vi "main.vi"() -> ()   [LabVIEW 2014]
uses:
  select.ctl
  Data.ctl
  <vilib>/Utility/miscctls.llb/LVBoundsTypeDef.ctl
panel:
  out "9":picture
  out "8":picture
  out "7":picture
  out "6":picture
  out "5":picture
  out "4":picture
  out "3":picture
  out "2":picture
  out "1":picture
  out "zero":picture
  out "ResultsAcumulado":string[][][](array[string])
  out "Listbox":i32(listbox)
  in  "Choose":string(combo)="luck"
  in  "Name":string
  in  "Exit":bool
  in  "Go":bool
  in  "ErrorIn":errorcluster
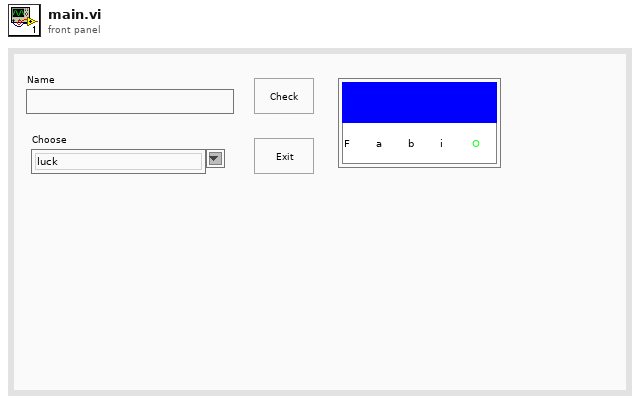
[diagram p1: front panel]
types:
  T1 = typedef "Data.ctl" = cluster{"Name":string, "Singles&Doubles":string[], "Results":string[][], "SinglesInOrder":string[], "DoublesInOrder":string[], "Option":string, "AllLetters":string[], "ByLuck":string, "SIndex":string[], "DIndex":string[], "ListOfNames":string[], "Cycles":cluster{"Laps":i32, "Counter":i32}, "Array":cluster{"AllLetters":string[], "ByLuck":string, "Option":string}[], "all":string[][], "all 2":string[][][], "WhichAndWhere":i32[], "Array 2":cluster{"AllLetters":string[], "ByLuck":string}[], "Chosen":string, "OptionForLuck":string, "ResultsAcumulado":string[][][]}
  T2 = typedef "select.ctl" = enum16{"init", "idle", "Segregate", "Select", "Singles&Doubles", "SearchForElements", "Display", "PutInOrder", "OptionToSelect", "Selected", "ChooseByLuck", "PrepareToShowByLuck", "PrepareToShowSelected", "Show", "ShowOnce"}
  T3 = cluster{"AllLetters":string[], "ByLuck":string}[]
  T4 = cluster{"AllLetters":string[], "ByLuck":string, "Option":string}[]
  T5 = typedef "LVBoundsTypeDef.ctl" = cluster{"Width":u32, "Height":u32}
  T6 = typedef "imagedata.ctl" = cluster{"image type":i32, "image depth":i32, "image":u8[], "mask":u8[], "colors":u32[], "Rectangle":cluster{"left":i16, "top":i16, "right":i16, "bottom":i16}}
  T7 = cluster{"AllLetters":string[], "ByLuck":string, "OptionForLuck":string}
  T8 = cluster{"AllLetters":string[], "ByLuck":string, "OptionForLuck":string}[]
  T9 = cluster{"AllLetters":string[], "Chosen":string}[]
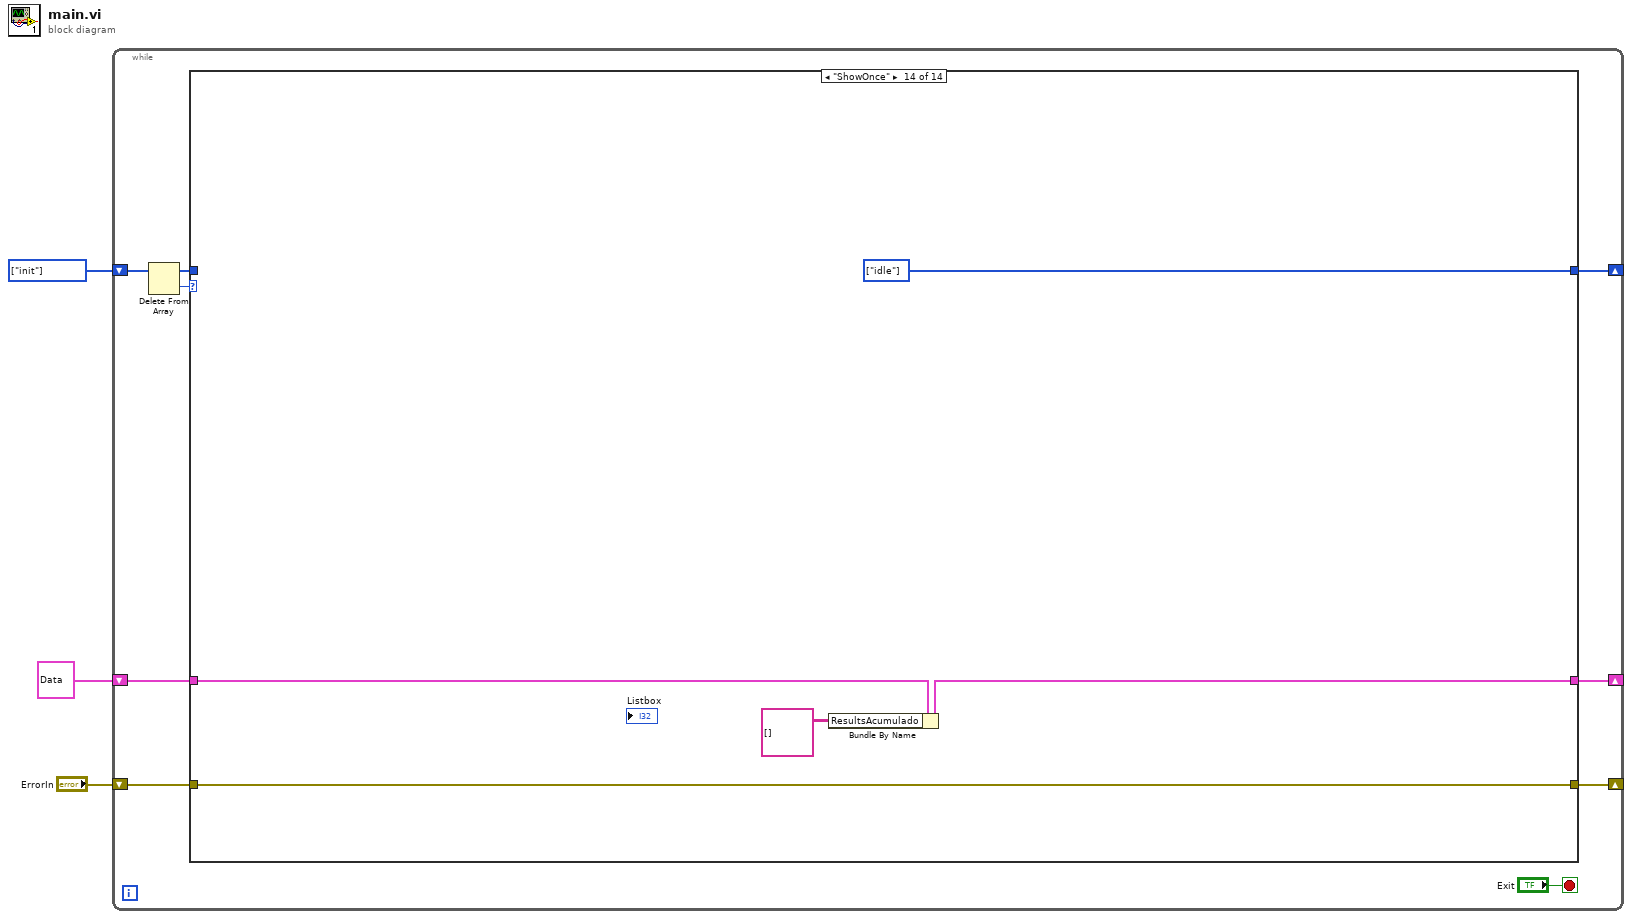
[diagram p0: block diagram]
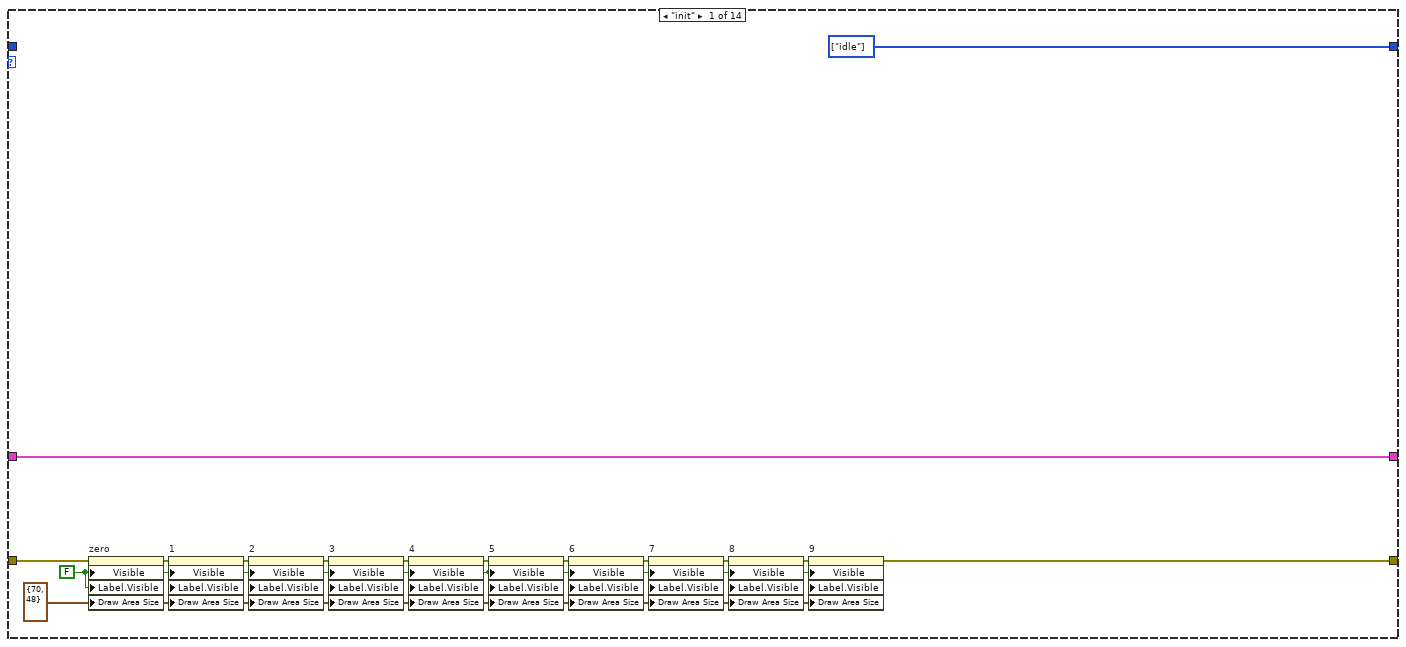
[diagram p2: hidden frame]
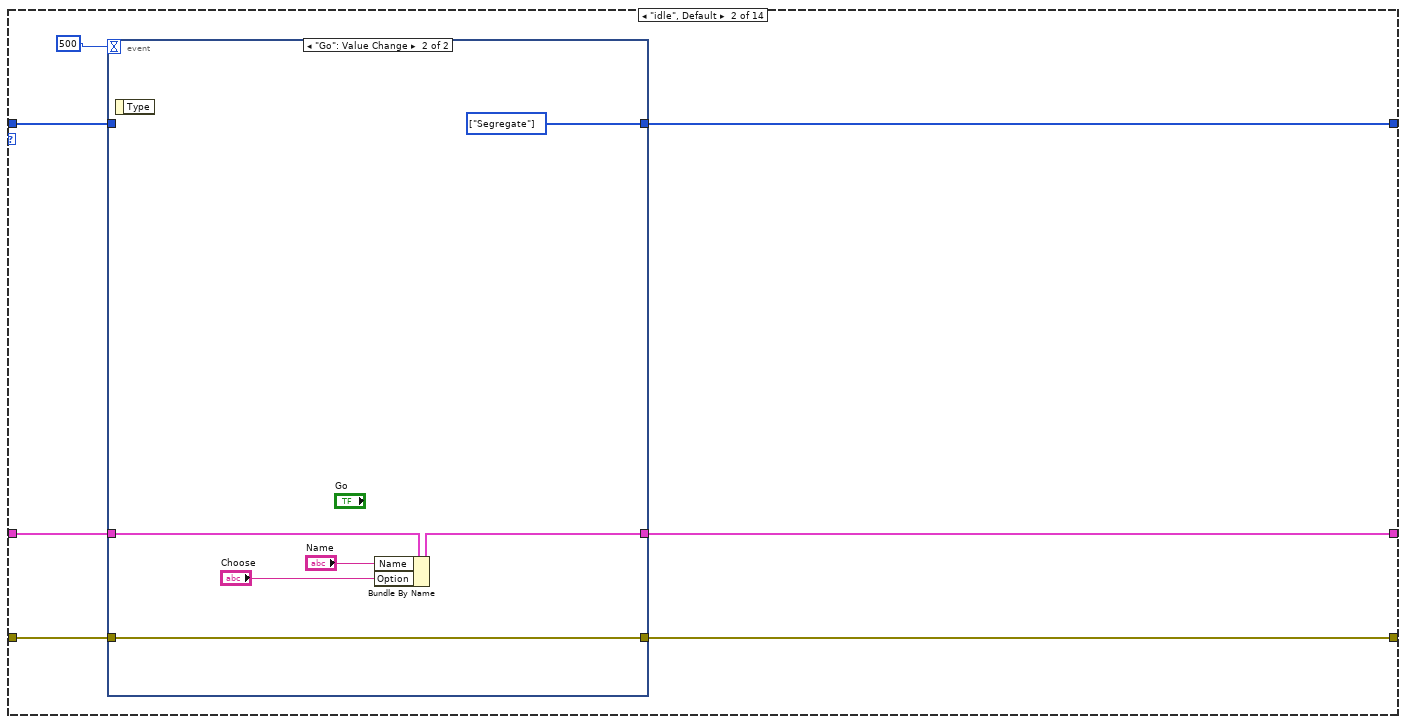
[diagram p3: hidden frame]
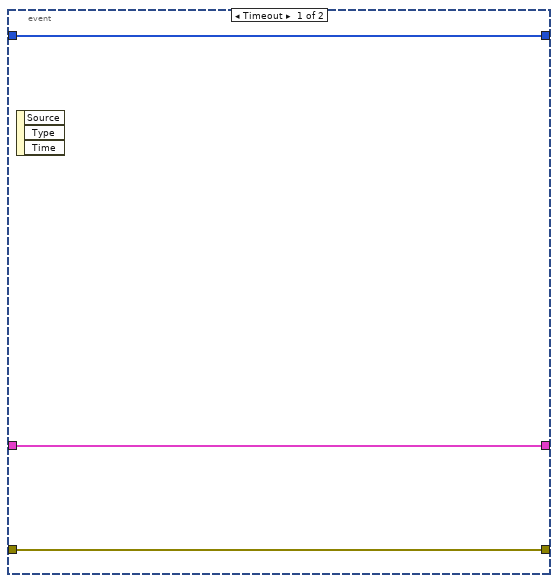
[diagram p4: hidden frame]
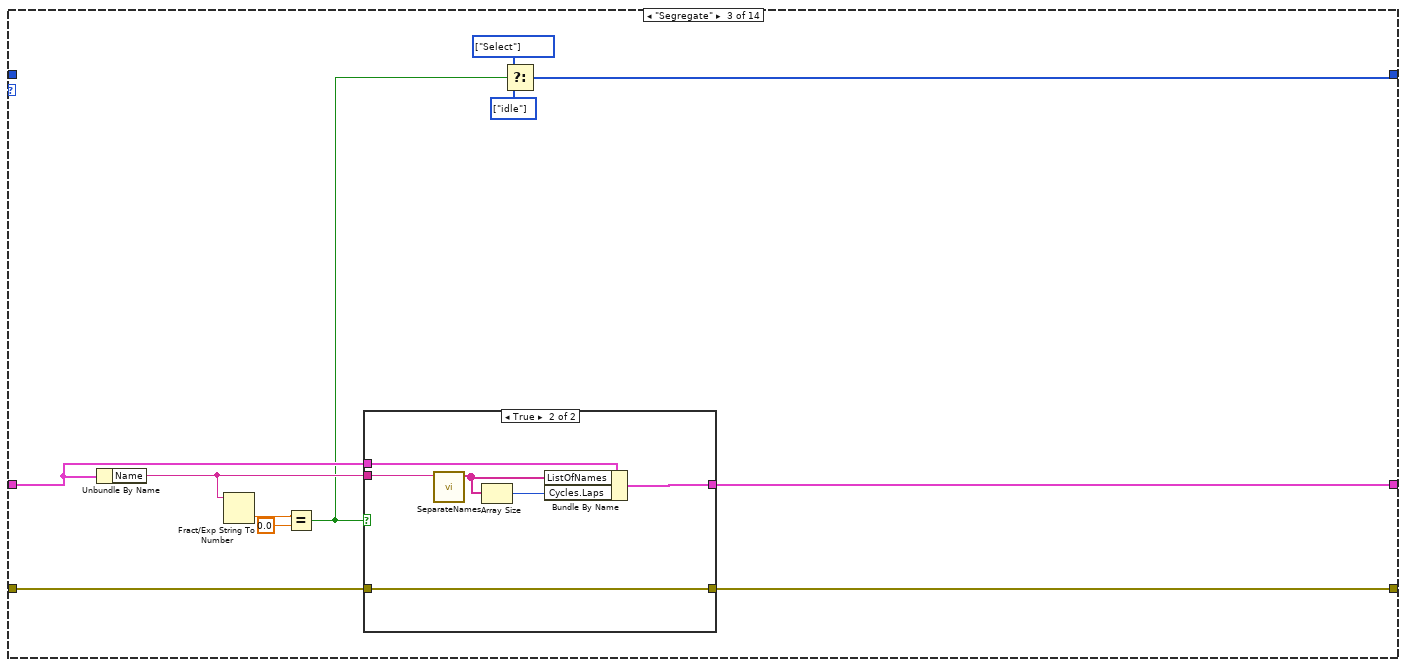
[diagram p5: hidden frame]
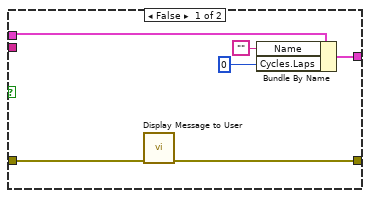
[diagram p6: hidden frame]
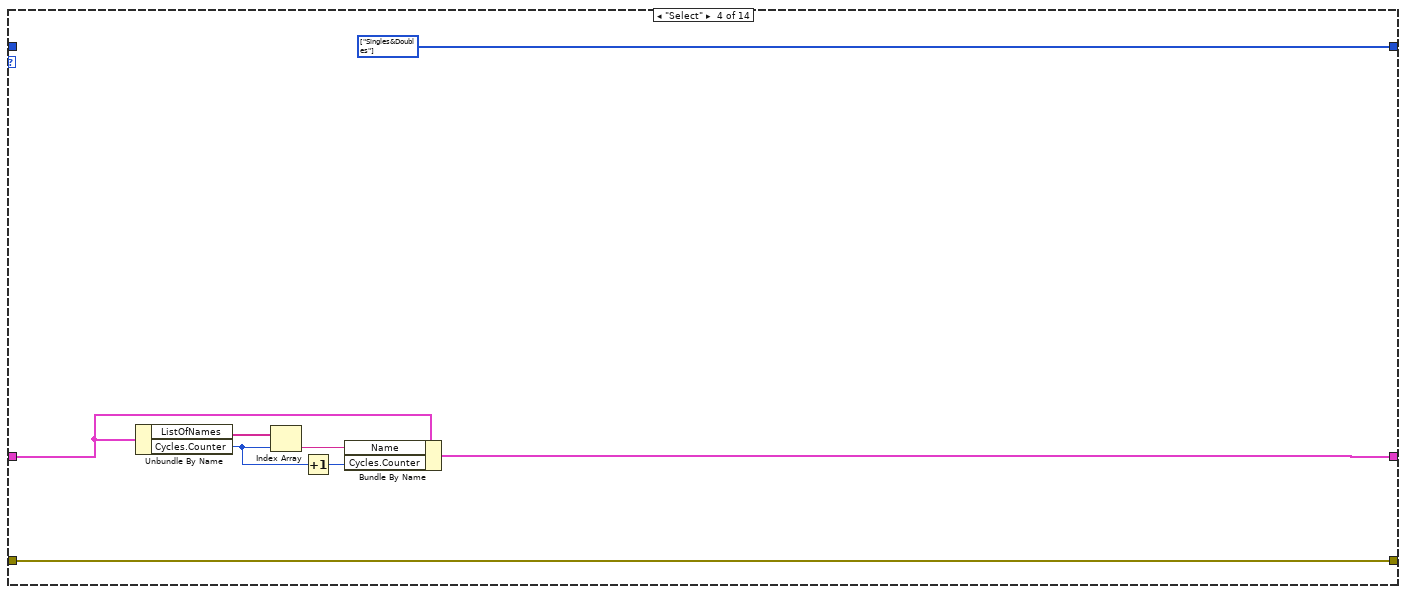
[diagram p7: hidden frame]
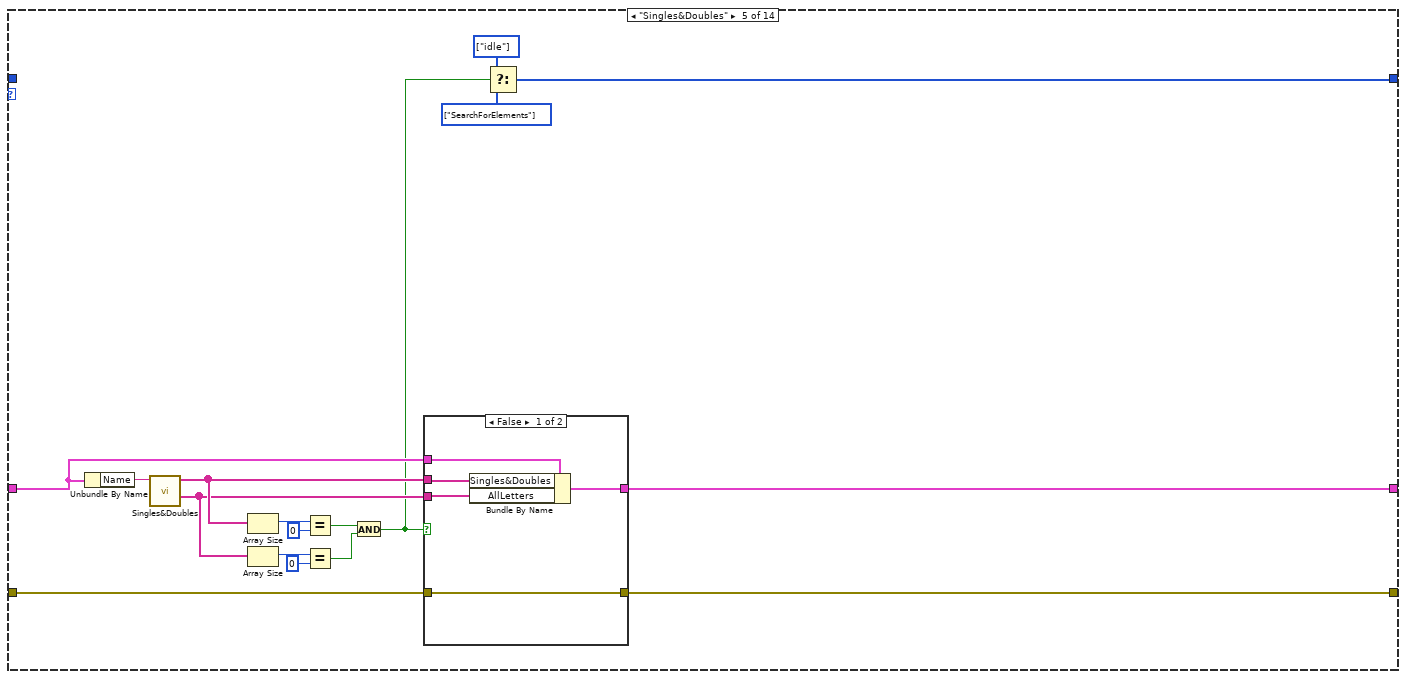
[diagram p8: hidden frame]
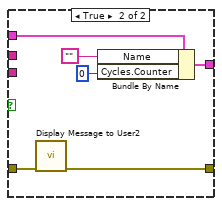
[diagram p9: hidden frame]
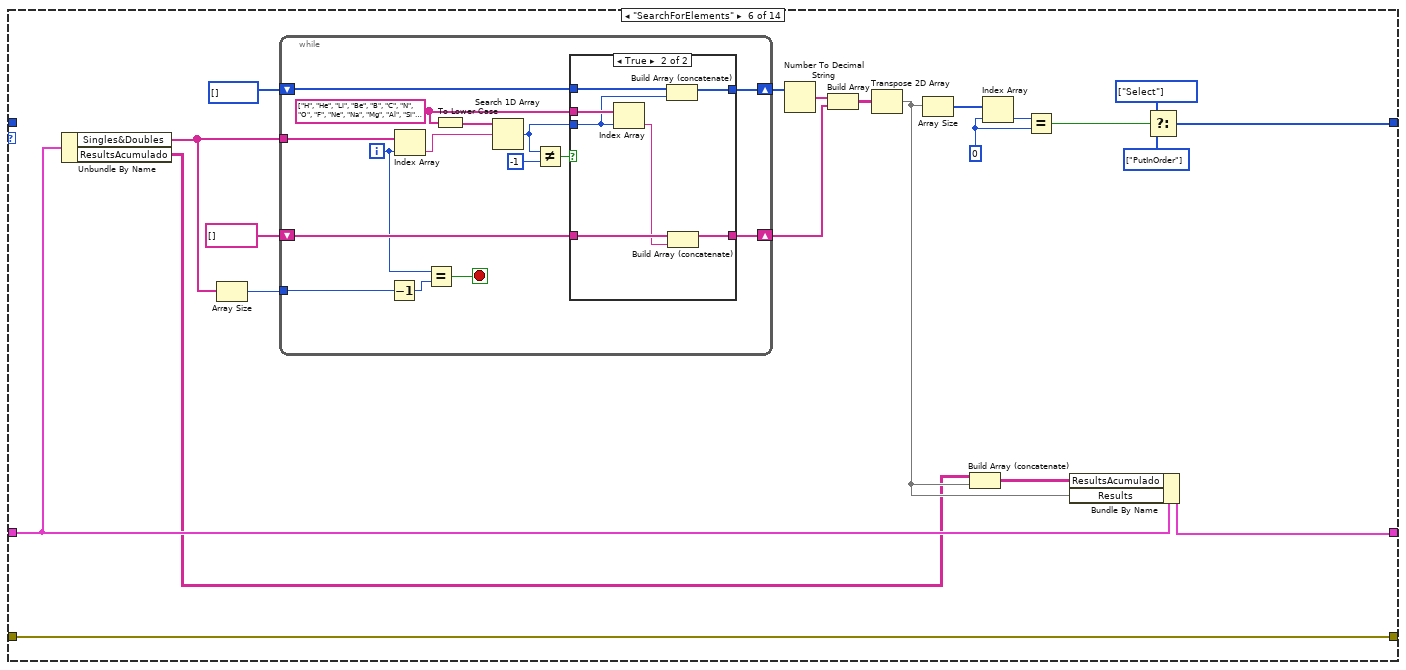
[diagram p10: hidden frame]
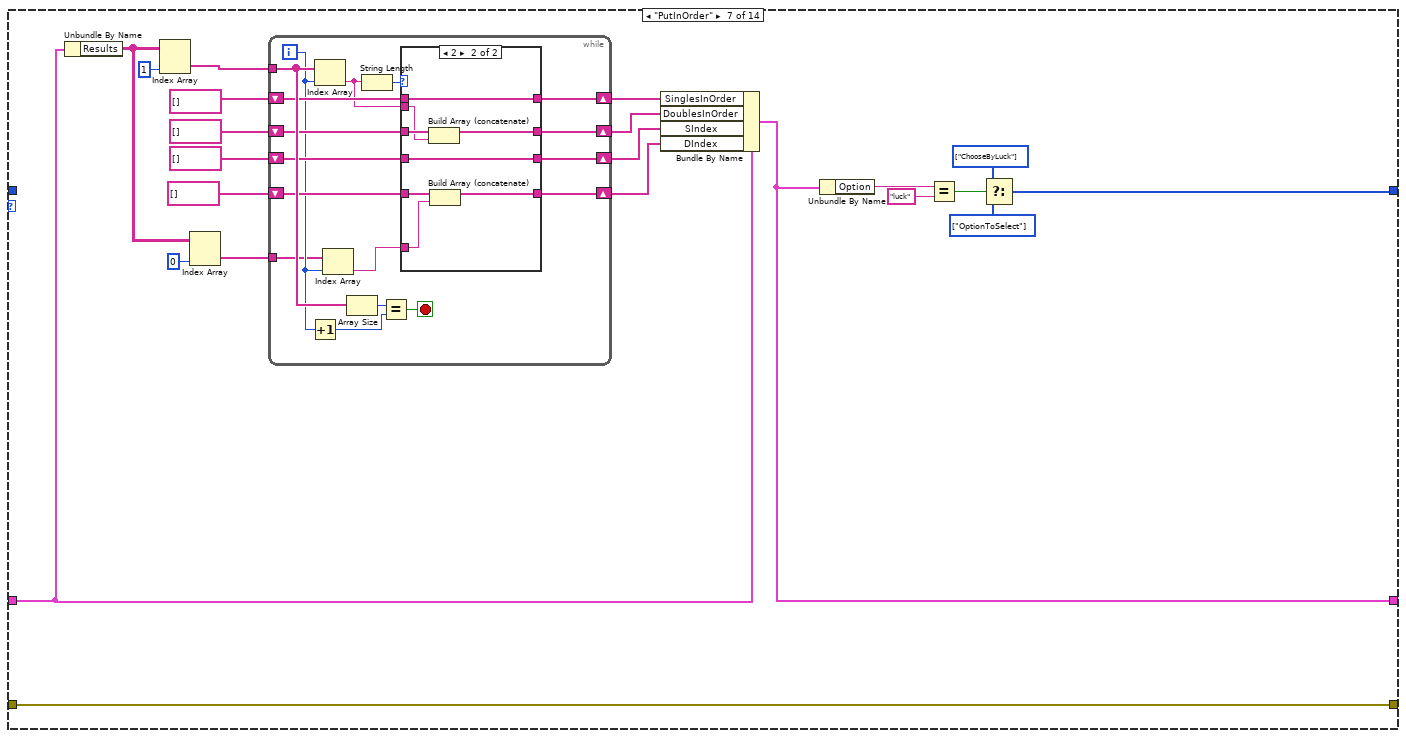
[diagram p12: hidden frame]
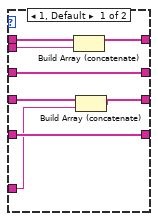
[diagram p13: hidden frame]
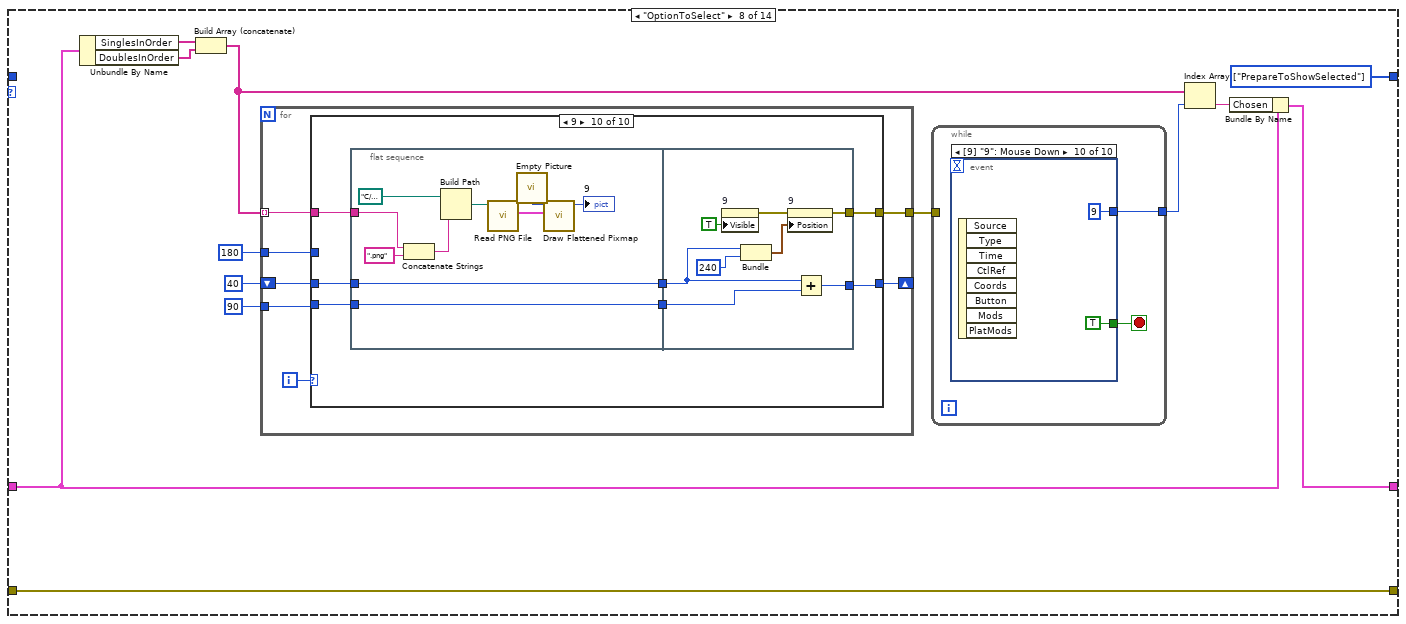
[diagram p14: hidden frame]
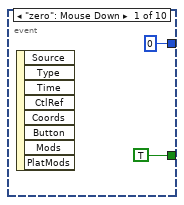
[diagram p15: hidden frame]
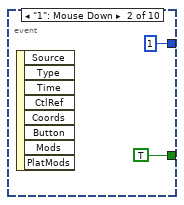
[diagram p16: hidden frame]
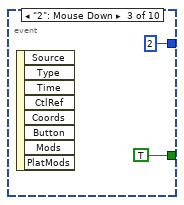
[diagram p17: hidden frame]
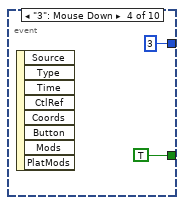
[diagram p18: hidden frame]
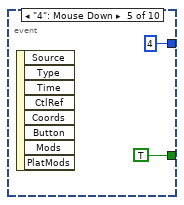
[diagram p19: hidden frame]
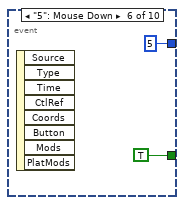
[diagram p20: hidden frame]
diagram:
  w3 = T2[] [enum."init"] items=["init", "idle", "Segregate", "Select", "Singles&Doubles", "SearchForElements", "Display", "PutInOrder", "OptionToSelect", "Selected", "ChooseByLuck", "PrepareToShowByLuck", "PrepareToShowSelected", "Show", "ShowOnce"]
  n1 = while {
    shift-right: [w9] -> _
    shift-left: w3 -> [w12]
    shift-right: [w7] -> _
    shift-left: T1 {"Name"="", "Singles&Doubles"=[], "Results"=[], "SinglesInOrder"=[], "DoublesInOrder"=[], "Option"="", "AllLetters"=[], "ByLuck"="", "SIndex"=[], "DIndex"=[], "ListOfNames"=[], "Cycles"={"Laps"=0, "Counter"=0}, "Array"=[], "all"=[], "all 2"=[], "WhichAndWhere"=[], "Array 2"=[], "Chosen"="", "OptionForLuck"="", "ResultsAcumulado"=[]} -> [w8]
    shift-right: [w6] -> _
    shift-left: "ErrorIn" -> [w5]
    stop <- "Exit" stop-if-true
    n2 = Delete From Array(array=w12) -> (deleted portion=w11:T2, array with subset deleted=w10:T2[])  [unwired: 2 in]
    n3 = case shown="\"ShowOnce\"" w11 {
      tunnel: w10 -> [_ w30 _ _ _ _ _ _ _ _ _ _ _ _]
      tunnel: [w14 w34 w48 w68 w75 w107 w154 w214 w505 w537 w553 w592 w626 w647] -> w9
      tunnel: w8 -> [w15 w33 w54 w73 w91 w120 w168 w211 w508 w536 w555 w588 w622 w646]
      tunnel: [w15 w32 w53 w69 w90 w119 w153 w210 w507 w535 w552 w584 w621 w645] -> w7
      tunnel: [w17 w28 w46 w67 w79 w123 w169 w215 w506 w540 w554 w601 w602 w643] -> w6
      tunnel: w5 -> [w16 w31 w47 w67 w80 w123 w169 w215 w506 w540 w554 w601 w612 w643]
      frame "init" {
        w13 = T5 {"Width"=70, "Height"=48} ("Bounds")
        w14 = T2[] [enum."idle"] items=["init", "idle", "Segregate", "Select", "Singles&Doubles", "SearchForElements", "Display", "PutInOrder", "OptionToSelect", "Selected", "ChooseByLuck", "PrepareToShowByLuck", "PrepareToShowSelected", "Show", "ShowOnce"] ("f")
        w18 = FALSE
        n4 = property on="zero" class="Pict"(error in=w16, "Visible"=w18, "Label.Visible"=w18, "Draw Area Size"=w13) -> (error out=w19:errorcluster)  [unwired: 1 in, 1 out]
        n5 = property on="1" class="Pict"(error in=w19, "Visible"=w18, "Label.Visible"=w18, "Draw Area Size"=w13) -> (error out=w20:errorcluster)  [unwired: 1 in, 1 out]
        n6 = property on="2" class="Pict"(error in=w20, "Visible"=w18, "Label.Visible"=w18, "Draw Area Size"=w13) -> (error out=w21:errorcluster)  [unwired: 1 in, 1 out]
        n7 = property on="3" class="Pict"(error in=w21, "Visible"=w18, "Label.Visible"=w18, "Draw Area Size"=w13) -> (error out=w22:errorcluster)  [unwired: 1 in, 1 out]
        n8 = property on="4" class="Pict"(error in=w22, "Visible"=w18, "Label.Visible"=w18, "Draw Area Size"=w13) -> (error out=w23:errorcluster)  [unwired: 1 in, 1 out]
        n9 = property on="5" class="Pict"(error in=w23, "Visible"=w18, "Label.Visible"=w18, "Draw Area Size"=w13) -> (error out=w24:errorcluster)  [unwired: 1 in, 1 out]
        n10 = property on="6" class="Pict"(error in=w24, "Visible"=w18, "Label.Visible"=w18, "Draw Area Size"=w13) -> (error out=w25:errorcluster)  [unwired: 1 in, 1 out]
        n11 = property on="7" class="Pict"(error in=w25, "Visible"=w18, "Label.Visible"=w18, "Draw Area Size"=w13) -> (error out=w26:errorcluster)  [unwired: 1 in, 1 out]
        n12 = property on="8" class="Pict"(error in=w26, "Visible"=w18, "Label.Visible"=w18, "Draw Area Size"=w13) -> (error out=w27:errorcluster)  [unwired: 1 in, 1 out]
        n13 = property on="9" class="Pict"(error in=w27, "Visible"=w18, "Label.Visible"=w18, "Draw Area Size"=w13) -> (error out=w17:errorcluster)  [unwired: 1 in, 1 out]
      }
      frame "idle", Default {
        n14 = event shown="[1] \"Go\": Value Change" {
          selector: _ -> [_ _]
          dyn-events: _ -> [_ _]
          timeout: 500 -> [_ _]
          tunnel: w30 -> [w37 _]
          tunnel: [w37 w42] -> w34
          tunnel: [w36 w40] -> w32
          tunnel: w33 -> [w36 w41]
          tunnel: [w35 w43] -> w28
          tunnel: w31 -> [w35 w43]
          event Timeout {
            n15 = event-data() -> ()  [unwired: 1 in, 3 out]
          }
          event "Go": Value Change {
            w42 = T2[] [enum."Segregate"] items=["init", "idle", "Segregate", "Select", "Singles&Doubles", "SearchForElements", "Display", "PutInOrder", "OptionToSelect", "Selected", "ChooseByLuck", "PrepareToShowByLuck", "PrepareToShowSelected", "Show", "ShowOnce"]
            n16 = event-data() -> ()  [unwired: 1 in, 1 out]
            n17 = Bundle By Name(cluster=w41, "Name"="Name", "Option"="Choose") -> (w40:T1)
          }
        }
      }
      frame "Segregate" {
        w45 = T2[] [enum."idle"] items=["init", "idle", "Segregate", "Select", "Singles&Doubles", "SearchForElements", "Display", "PutInOrder", "OptionToSelect", "Selected", "ChooseByLuck", "PrepareToShowByLuck", "PrepareToShowSelected", "Show", "ShowOnce"]
        w44 = T2[] [enum."Select"] items=["init", "idle", "Segregate", "Select", "Singles&Doubles", "SearchForElements", "Display", "PutInOrder", "OptionToSelect", "Selected", "ChooseByLuck", "PrepareToShowByLuck", "PrepareToShowSelected", "Show", "ShowOnce"]
        n18 = Unbundle By Name(w54) -> ("Name"=w52:string)
        n19 = Fract/Exp String To Number(string=w52) -> (number=w51:dbl)  [unwired: 3 in, 1 out]
        n20 = Equal?(x=w51, y=0.0) -> (x = y?=w49:bool)
        n21 = case shown="True" w49 {
          tunnel: w52 -> [_ w66]
          tunnel: w54 -> [w58 w65]
          tunnel: [w57 w62] -> w53
          tunnel: w47 -> [w60 w61]
          tunnel: [w59 w61] -> w46
          frame False {
            n22 = call "Display Message to User"("error in (no error)"=w60) -> ("error out"=w59:errorcluster)  [unwired: 9 in, 1 out]
            n23 = Bundle By Name(cluster=w58, "Name"="", "Cycles.Laps"=0) -> (w57:T1)
          }
          frame True {
            n24 = call "SeparateNames.vi"("CompleteName"=w66) -> ("SeparateWords"=w63:string[])  [unwired: 10 in]
            n25 = Array Size(array=w63) -> (size(s)=w64:i32)
            n26 = Bundle By Name(cluster=w65, "ListOfNames"=w63, "Cycles.Laps"=w64) -> (w62:T1)
          }
        }
        n27 = Select(t=w44, s=w49, f=w45) -> (s? t:f=w48:T2[])
      }
      frame "Select" {
        w68 = T2[] [enum."Singles&Doubles"] items=["init", "idle", "Segregate", "Select", "Singles&Doubles", "SearchForElements", "Display", "PutInOrder", "OptionToSelect", "Selected", "ChooseByLuck", "PrepareToShowByLuck", "PrepareToShowSelected", "Show", "ShowOnce"]
        n28 = Unbundle By Name(w73) -> ("ListOfNames"=w74:string[], "Cycles.Counter"=w71:i32)
        n29 = Index Array(array=w74, index=w71) -> (element=w70:string)
        n30 = Increment(x=w71) -> (x+1=w72:i32)
        n31 = Bundle By Name(cluster=w73, "Name"=w70, "Cycles.Counter"=w72) -> (w69:T1)
      }
      frame "Singles&Doubles" {
        w76 = T2[] [enum."idle"] items=["init", "idle", "Segregate", "Select", "Singles&Doubles", "SearchForElements", "Display", "PutInOrder", "OptionToSelect", "Selected", "ChooseByLuck", "PrepareToShowByLuck", "PrepareToShowSelected", "Show", "ShowOnce"]
        w77 = T2[] [enum."SearchForElements"] items=["init", "idle", "Segregate", "Select", "Singles&Doubles", "SearchForElements", "Display", "PutInOrder", "OptionToSelect", "Selected", "ChooseByLuck", "PrepareToShowByLuck", "PrepareToShowSelected", "Show", "ShowOnce"]
        n32 = Unbundle By Name(w91) -> ("Name"=w89:string)
        n33 = call "Singles&Doubles.vi"("Name"=w89) -> ("AllLetters"=w87:string[], "Singles&Doubles"=w88:string[])  [unwired: 9 in]
        n34 = Array Size(array=w88) -> (size(s)=w86:i32)
        n35 = Array Size(array=w87) -> (size(s)=w85:i32)
        n36 = Equal?(x=w86, y=0) -> (x = y?=w82:bool)
        n37 = Equal?(x=w85, y=0) -> (x = y?=w81:bool)
        n38 = And(x=w82, y=w81) -> (x .and. y?=w78:bool)
        n39 = case shown="False" w78 {
          tunnel: w91 -> [w96 w100]
          tunnel: [w95 w99] -> w90
          tunnel: w88 -> [w94 _]
          tunnel: w87 -> [w93 _]
          tunnel: w80 -> [w92 w102]
          tunnel: [w92 w101] -> w79
          frame False {
            n40 = Bundle By Name(cluster=w96, "Singles&Doubles"=w94, "AllLetters"=w93) -> (w95:T1)
          }
          frame True {
            n41 = call "Display Message to User2"("error in (no error)"=w102) -> ("error out"=w101:errorcluster)  [unwired: 9 in, 1 out]
            n42 = Bundle By Name(cluster=w100, "Name"="", "Cycles.Counter"=0) -> (w99:T1)
          }
        }
        n43 = Select(t=w76, s=w78, f=w77) -> (s? t:f=w75:T2[])
      }
      frame "SearchForElements" {
        w106 = T2[] [enum."Select"] items=["init", "idle", "Segregate", "Select", "Singles&Doubles", "SearchForElements", "Display", "PutInOrder", "OptionToSelect", "Selected", "ChooseByLuck", "PrepareToShowByLuck", "PrepareToShowSelected", "Show", "ShowOnce"] ("t")
        w110 = 0
        w108 = T2[] [enum."PutInOrder"] items=["init", "idle", "Segregate", "Select", "Singles&Doubles", "SearchForElements", "Display", "PutInOrder", "OptionToSelect", "Selected", "ChooseByLuck", "PrepareToShowByLuck", "PrepareToShowSelected", "Show", "ShowOnce"]
        n44 = Unbundle By Name(w120) -> ("Singles&Doubles"=w118:string[], "ResultsAcumulado"=w103:string[][][])
        n45 = Array Size(array=w118) -> (size(s)=w121:i32)
        n46 = while {
          tunnel: w118 -> [w133]
          shift-right: [w135] -> w114
          shift-left: string[] [] -> [w134]
          tunnel: w121 -> [w127]
          shift-right: [w125] -> w113
          shift-left: i32[] [] -> [w124]
          i -> [w131]
          stop <- w130 stop-if-true
          w126 = string[] ["H", "He", "Li", "Be", "B", "C", "N", "O", "F", "Ne", "Na", "Mg", "Al", "Si", "P", "S", "Cl", "Ar", "K", "Ca", "Sc", "Ti", "V", "Cr", "Mn", "Fe", "Co", "Ni", "Cu", "Zn", "Ga", "Ge", "As", "Se", "Br", "Kr", "Rb", "Sr", "Y", "Zr", "Nb", "Mo", "Tc", "Ru", "Rh", "Pd", "Ag", "Cd", "In", "Sn", "Sb", "Te", "I", "Xe", "Cs", "Ba", "La", "Ce", "Pr", "Nd", "Pm", "Sm", "Eu", "Gd", "Tb", "Dy", "Ho", "Er", "Tm", "Yb", "Lu", "Hf", "Ta", "W", "Re", "Os", "Ir", "Pt", "Au", "Hg", "Tl", "Pb", "Bi", "Po", "At", "Rn", "Fr", "Ra", "Ac", "Th", "Pa", "U", "Np", "Pu", "Am", "Cm", "Bk", "Cf", "Es", "Fm", "Md", "No", "Lr", "Rf", "Db", "Sg", "Bh", "Hs", "Mt"]
          n47 = Decrement(x=w127) -> (x-1=w128:i32)
          n48 = Index Array(array=w133, index=w131) -> (element=w138:string)
          n49 = Equal?(x=w131, y=w128) -> (x = y?=w130:bool)
          n50 = To Lower Case(string=w126) -> (all lower case string=w129:string[])
          n51 = Search 1D Array(1D array=w129, element=w138) -> (index of element=w132:i32)  [unwired: 1 in]
          n52 = Not Equal?(x=w132, y=-1) -> (x != y?=w136:bool)
          n53 = case shown="True" w136 {
            tunnel: [w140 w144] -> w135
            tunnel: w134 -> [w140 w147]
            tunnel: w126 -> [_ w146]
            tunnel: w132 -> [_ w141]
            tunnel: [w139 w143] -> w125
            tunnel: w124 -> [w139 w142]
            frame False {
            }
            frame True {
              n54 = Index Array(array=w146, index=w141) -> (element=w145:string)
              n55 = Build Array (concatenate)(w142, w141) -> (w143:i32[])
              n56 = Build Array (concatenate)(w147, w145) -> (w144:string[])
            }
          }
        }
        n57 = Number To Decimal String(number=w113) -> (decimal integer string=w116:string[])  [unwired: 1 in]
        n58 = Build Array(w116, w114) -> (w115:string[][])
        n59 = Transpose 2D Array(2D array=w115) -> (transposed array=w104:string[][])
        n60 = Array Size(array=w104) -> (size(s)=w112:i32[])
        n61 = Build Array (concatenate)(w103, w104) -> (w105:string[][][])
        n62 = Index Array(array=w112, index=w110) -> (element=w111:i32)
        n63 = Equal?(x=w111, y=w110) -> (x = y?=w109:bool)
        n64 = Bundle By Name(cluster=w120, "ResultsAcumulado"=w105, "Results"=w104) -> (w119:T1)
        n65 = Select(t=w106, s=w109, f=w108) -> (s? t:f=w107:T2[])
      }
      frame "PutInOrder" {
        w149 = T2[] [enum."OptionToSelect"] items=["init", "idle", "Segregate", "Select", "Singles&Doubles", "SearchForElements", "Display", "PutInOrder", "OptionToSelect", "Selected", "ChooseByLuck", "PrepareToShowByLuck", "PrepareToShowSelected", "Show", "ShowOnce"]
        w150 = T2[] [enum."ChooseByLuck"] items=["init", "idle", "Segregate", "Select", "Singles&Doubles", "SearchForElements", "Display", "PutInOrder", "OptionToSelect", "Selected", "ChooseByLuck", "PrepareToShowByLuck", "PrepareToShowSelected", "Show", "ShowOnce"]
        n66 = Unbundle By Name(w168) -> ("Results"=w156:string[][])
        n67 = Index Array(array=w156, index (col)=1 ("disabled index (col)")) -> (element=w158:string[])  [unwired: 1 in]
        n68 = Index Array(array=w156, index (col)=0 ("disabled index (col)")) -> (element=w155:string[])  [unwired: 1 in]
        n69 = while {
          tunnel: w158 -> [w186]
          shift-right: [w183] -> w165
          shift-left: string[] [] -> [w182]
          shift-right: [w180] -> w164
          shift-left: string[] [] -> [w181]
          shift-right: [w178] -> w161
          shift-left: string[] [] -> [w179]
          shift-right: [w176] -> w160
          shift-left: string[] [] -> [w177]
          tunnel: w155 -> [w173]
          i -> [w174]
          stop <- w171 stop-if-true
          n70 = Increment(x=w174) -> (x+1=w184:i32)
          n71 = Index Array(array=w186, index=w174) -> (element=w175:string)
          n72 = Index Array(array=w173, index=w174) -> (element=w172:string)
          n73 = Array Size(array=w186) -> (size(s)=w185:i32)
          n74 = String Length(string=w175) -> (length=w170:i32)
          n75 = Equal?(x=w185, y=w184) -> (x = y?=w171:bool)
          n76 = case shown="2" w170 {
            tunnel: [w192 w202] -> w183
            tunnel: w182 -> [w194 w202]
            tunnel: w181 -> [w193 w200]
            tunnel: [w193 w201] -> w180
            tunnel: w179 -> [w191 w197]
            tunnel: [w190 w197] -> w178
            tunnel: w177 -> [w189 w198]
            tunnel: [w189 w199] -> w176
            tunnel: w175 -> [w188 w196]
            tunnel: w172 -> [w187 w195]
            frame 1, Default {
              n77 = Build Array (concatenate)(w194, w188) -> (w192:string[])
              n78 = Build Array (concatenate)(w191, w187) -> (w190:string[])
            }
            frame 2 {
              n79 = Build Array (concatenate)(w200, w196) -> (w201:string[])
              n80 = Build Array (concatenate)(w198, w195) -> (w199:string[])
            }
          }
        }
        n81 = Bundle By Name(cluster=w168, "SinglesInOrder"=w165, "DoublesInOrder"=w164, "SIndex"=w161, "DIndex"=w160) -> (w153:T1)
        n82 = Unbundle By Name(w153) -> ("Option"=w152:string)
        n83 = Equal?(x=w152, y="luck") -> (x = y?=w148:bool)
        n84 = Select(t=w150, s=w148, f=w149) -> (s? t:f=w154:T2[])
      }
      frame "OptionToSelect" {
        w214 = T2[] [enum."PrepareToShowSelected"] items=["init", "idle", "Segregate", "Select", "Singles&Doubles", "SearchForElements", "Display", "PutInOrder", "OptionToSelect", "Selected", "ChooseByLuck", "PrepareToShowByLuck", "PrepareToShowSelected", "Show", "ShowOnce"] ("f")
        n85 = Unbundle By Name(w211) -> ("SinglesInOrder"=w213:string[], "DoublesInOrder"=w212:string[])
        n86 = Build Array (concatenate)(w213, w212) -> (w204:string[])
        n87 = for {
          tunnel: w204 -> [w239] mode=indexing
          shift-right: [w243] -> _
          shift-left: 40 -> [w244]
          tunnel: 90 ("y") -> [w241]
          tunnel: [w240] -> w206
          tunnel: 180 -> [w238]
          i -> [w242]
          n88 = case shown="9" w242 {
            tunnel: w239 -> [w252 w280 w308 w336 w364 w389 w411 w434 w459 w485]
            tunnel: w244 -> [w251 w279 w307 w335 w363 _ _ w433 w458 w484]
            tunnel: [w250 w278 w306 w334 w362 w388 w410 w432 w457 w483] -> w243
            tunnel: w241 -> [w248 w276 w305 w333 w361 w387 w409 w431 w456 w482]
            tunnel: [w247 w275 w303 w331 w359 w385 w407 w429 w454 w480] -> w240
            tunnel: w238 -> [w245 w273 w302 w330 w358 _ _ _ _ _]
            frame 0, Default {
              n89 = flat-sequence {
                tunnel: w252 -> [w257]
                tunnel: [w259] -> w253
                tunnel: w251 -> [w259]
                tunnel: [w255] -> w249
                tunnel: w248 -> [w255]
                tunnel: [w254] -> w246
                tunnel: w245 -> [w254]
                tunnel: w253 -> [w266]
                tunnel: [w271] -> w250
                tunnel: w249 -> [w270]
                tunnel: [w269] -> w247
                tunnel: w246 -> [w265]
                frame #0 {
                  n90 = Concatenate Strings(w257, ".png" ("string")) -> (w258:string)
                  n91 = Build Path(base path=path "C:/Users/beck.to.beck/Documents/LabVIEW Data/BrBa/elements", name or relative path=w258) -> (appended path=w262:path)
                  n92 = call <vilib>:"Read PNG File.vi"("path to PNG file"=w262) -> ("image data"=w261:T6)  [unwired: 8 in, 2 out]
                  n93 = call "Empty Picture"() -> ("empty picture"=w263:picture)
                  n94 = call <vilib>:"Draw Flattened Pixmap.vi"("image data"=w261, "picture"=w263) -> ("new picture"=→"zero":picture)  [unwired: 7 in]
                }
                frame #1 {
                  n95 = property on="zero" class="Pict"("Visible"=TRUE) -> (error out=w267:errorcluster)  [unwired: 2 in, 1 out]
                  n96 = Bundle(w266, w265) -> (w272:cluster{i32, i32})  [unwired: 1 in]
                  n97 = property on="zero" class="Pict"(error in=w267, "Position"=w272) -> (error out=w269:errorcluster)  [unwired: 1 in, 1 out]
                  n98 = Add(x=w266, y=w270) -> (x+y=w271:i32)
                }
              }
            }
            frame 1 {
              n99 = flat-sequence {
                tunnel: w280 -> [w285]
                tunnel: [w287] -> w281
                tunnel: w279 -> [w287]
                tunnel: [w283] -> w277
                tunnel: w276 -> [w283]
                tunnel: [w282] -> w274
                tunnel: w273 -> [w282]
                tunnel: w281 -> [w295]
                tunnel: [w299] -> w278
                tunnel: w277 -> [w298]
                tunnel: [w297] -> w275
                tunnel: w274 -> [w294]
                frame #0 {
                  n100 = Concatenate Strings(w285, ".png" ("string")) -> (w284:string)
                  n101 = Build Path(base path=path "C:/Users/beck.to.beck/Documents/LabVIEW Data/BrBa/elements", name or relative path=w284) -> (appended path=w290:path)
                  n102 = call <vilib>:"Read PNG File.vi"("path to PNG file"=w290) -> ("image data"=w289:T6)  [unwired: 8 in, 2 out]
                  n103 = call "Empty Picture"() -> ("empty picture"=w291:picture)
                  n104 = call <vilib>:"Draw Flattened Pixmap.vi"("image data"=w289, "picture"=w291) -> ("new picture"=→"1":picture)  [unwired: 7 in]
                }
                frame #1 {
                  n105 = property on="1" class="Pict"("Visible"=TRUE) -> (error out=w293:errorcluster)  [unwired: 2 in, 1 out]
                  n106 = Bundle(w295, w294) -> (w300:cluster{i32, i32})  [unwired: 1 in]
                  n107 = property on="1" class="Pict"(error in=w293, "Position"=w300) -> (error out=w297:errorcluster)  [unwired: 1 in, 1 out]
                  n108 = Add(x=w295, y=w298) -> (x+y=w299:i32)
                }
              }
            }
            frame 2 {
              n109 = flat-sequence {
                tunnel: w308 -> [w313]
                tunnel: [w315] -> w309
                tunnel: w307 -> [w315]
                tunnel: w305 -> [w311]
                tunnel: [w311] -> w304
                tunnel: w302 -> [w310]
                tunnel: [w310] -> w301
                tunnel: w309 -> [w323]
                tunnel: [w327] -> w306
                tunnel: w304 -> [w326]
                tunnel: [w325] -> w303
                tunnel: w301 -> [w321]
                frame #0 {
                  n110 = Concatenate Strings(w313, ".png" ("string")) -> (w312:string)
                  n111 = Build Path(base path=path "C:/Users/beck.to.beck/Documents/LabVIEW Data/BrBa/elements", name or relative path=w312) -> (appended path=w318:path)
                  n112 = call <vilib>:"Read PNG File.vi"("path to PNG file"=w318) -> ("image data"=w317:T6)  [unwired: 8 in, 2 out]
                  n113 = call "Empty Picture"() -> ("empty picture"=w319:picture)
                  n114 = call <vilib>:"Draw Flattened Pixmap.vi"("image data"=w317, "picture"=w319) -> ("new picture"=→"2":picture)  [unwired: 7 in]
                }
                frame #1 {
                  n115 = property on="2" class="Pict"("Visible"=TRUE) -> (error out=w322:errorcluster)  [unwired: 2 in, 1 out]
                  n116 = Bundle(w323, w321) -> (w328:cluster{i32, i32})  [unwired: 1 in]
                  n117 = property on="2" class="Pict"(error in=w322, "Position"=w328) -> (error out=w325:errorcluster)  [unwired: 1 in, 1 out]
                  n118 = Add(x=w323, y=w326) -> (x+y=w327:i32)
                }
              }
            }
            frame 3 {
              n119 = flat-sequence {
                tunnel: w336 -> [w341]
                tunnel: [w343] -> w337
                tunnel: w335 -> [w343]
                tunnel: w333 -> [w339]
                tunnel: [w339] -> w332
                tunnel: w330 -> [w338]
                tunnel: [w338] -> w329
                tunnel: w337 -> [w351]
                tunnel: [w355] -> w334
                tunnel: w332 -> [w354]
                tunnel: [w353] -> w331
                tunnel: w329 -> [w350]
                frame #0 {
                  n120 = Concatenate Strings(w341, ".png" ("string")) -> (w340:string)
                  n121 = Build Path(base path=path "C:/Users/beck.to.beck/Documents/LabVIEW Data/BrBa/elements", name or relative path=w340) -> (appended path=w346:path)
                  n122 = call <vilib>:"Read PNG File.vi"("path to PNG file"=w346) -> ("image data"=w345:T6)  [unwired: 8 in, 2 out]
                  n123 = call "Empty Picture"() -> ("empty picture"=w347:picture)
                  n124 = call <vilib>:"Draw Flattened Pixmap.vi"("image data"=w345, "picture"=w347) -> ("new picture"=→"3":picture)  [unwired: 7 in]
                }
                frame #1 {
                  n125 = property on="3" class="Pict"("Visible"=TRUE) -> (error out=w349:errorcluster)  [unwired: 2 in, 1 out]
                  n126 = Bundle(w351, w350) -> (w356:cluster{i32, i32})  [unwired: 1 in]
                  n127 = property on="3" class="Pict"(error in=w349, "Position"=w356) -> (error out=w353:errorcluster)  [unwired: 1 in, 1 out]
                  n128 = Add(x=w351, y=w354) -> (x+y=w355:i32)
                }
              }
            }
            frame 4 {
              n129 = flat-sequence {
                tunnel: w364 -> [w369]
                tunnel: [w371] -> w365
                tunnel: w363 -> [w371]
                tunnel: w361 -> [w367]
                tunnel: [w367] -> w360
                tunnel: w358 -> [w366]
                tunnel: [w366] -> w357
                tunnel: w365 -> [w380]
                tunnel: [w384] -> w362
                tunnel: w360 -> [w383]
                tunnel: [w382] -> w359
                tunnel: w357 -> [w377]
                frame #0 {
                  n130 = Concatenate Strings(w369, ".png" ("string")) -> (w368:string)
                  n131 = Build Path(base path=path "C:/Users/beck.to.beck/Documents/LabVIEW Data/BrBa/elements", name or relative path=w368) -> (appended path=w374:path)
                  n132 = call <vilib>:"Read PNG File.vi"("path to PNG file"=w374) -> ("image data"=w373:T6)  [unwired: 8 in, 2 out]
                  n133 = call "Empty Picture"() -> ("empty picture"=w375:picture)
                  n134 = call <vilib>:"Draw Flattened Pixmap.vi"("image data"=w373, "picture"=w375) -> ("new picture"=→"4":picture)  [unwired: 7 in]
                }
                frame #1 {
                  n135 = property on="4" class="Pict"("Visible"=TRUE) -> (error out=w378:errorcluster)  [unwired: 2 in, 1 out]
                  n136 = Bundle(w380, w377) -> (w379:cluster{i32, i32})  [unwired: 1 in]
                  n137 = property on="4" class="Pict"(error in=w378, "Position"=w379) -> (error out=w382:errorcluster)  [unwired: 1 in, 1 out]
                  n138 = Add(x=w380, y=w383) -> (x+y=w384:i32)
                }
              }
            }
            frame 5 {
              n139 = flat-sequence {
                tunnel: w389 -> [w392]
                tunnel: w387 -> [w390]
                tunnel: [w390] -> w386
                tunnel: [w405] -> w388
                tunnel: w386 -> [w404]
                tunnel: [w403] -> w385
                frame #0 {
                  n140 = Concatenate Strings(w392, ".png" ("string")) -> (w391:string)
                  n141 = Build Path(base path=path "C:/Users/beck.to.beck/Documents/LabVIEW Data/BrBa/elements", name or relative path=w391) -> (appended path=w396:path)
                  n142 = call <vilib>:"Read PNG File.vi"("path to PNG file"=w396) -> ("image data"=w395:T6)  [unwired: 8 in, 2 out]
                  n143 = call "Empty Picture"() -> ("empty picture"=w397:picture)
                  n144 = call <vilib>:"Draw Flattened Pixmap.vi"("image data"=w395, "picture"=w397) -> ("new picture"=→"5":picture)  [unwired: 7 in]
                }
                frame #1 {
                  w401 = 40
                  n145 = property on="5" class="Pict"("Visible"=TRUE) -> (error out=w399:errorcluster)  [unwired: 2 in, 1 out]
                  n146 = Bundle(w401, 240) -> (w406:cluster{i32, i32})  [unwired: 1 in]
                  n147 = property on="5" class="Pict"(error in=w399, "Position"=w406) -> (error out=w403:errorcluster)  [unwired: 1 in, 1 out]
                  n148 = Add(x=w401, y=w404) -> (x+y=w405:i32)
                }
              }
            }
            frame 6 {
              n149 = flat-sequence {
                tunnel: w411 -> [w414]
                tunnel: w409 -> [w412]
                tunnel: [w412] -> w408
                tunnel: [w428] -> w410
                tunnel: w408 -> [w427]
                tunnel: [w426] -> w407
                frame #0 {
                  n150 = Concatenate Strings(w414, ".png" ("string")) -> (w413:string)
                  n151 = Build Path(base path=path "C:/Users/beck.to.beck/Documents/LabVIEW Data/BrBa/elements", name or relative path=w413) -> (appended path=w418:path)
                  n152 = call <vilib>:"Read PNG File.vi"("path to PNG file"=w418) -> ("image data"=w417:T6)  [unwired: 8 in, 2 out]
                  n153 = call "Empty Picture"() -> ("empty picture"=w419:picture)
                  n154 = call <vilib>:"Draw Flattened Pixmap.vi"("image data"=w417, "picture"=w419) -> ("new picture"=→"6":picture)  [unwired: 7 in]
                }
                frame #1 {
                  w422 = 40
                  n155 = property on="6" class="Pict"("Visible"=TRUE) -> (error out=w421:errorcluster)  [unwired: 2 in, 1 out]
                  n156 = Bundle(w422, 240) -> (w423:cluster{i32, i32})  [unwired: 1 in]
                  n157 = property on="6" class="Pict"(error in=w421, "Position"=w423) -> (error out=w426:errorcluster)  [unwired: 1 in, 1 out]
                  n158 = Add(x=w422, y=w427) -> (x+y=w428:i32)
                }
              }
            }
            frame 7 {
              n159 = flat-sequence {
                tunnel: w434 -> [w438]
                tunnel: [w440] -> w435
                tunnel: w433 -> [w440]
                tunnel: w431 -> [w436]
                tunnel: [w436] -> w430
                tunnel: w435 -> [w448]
                tunnel: [w453] -> w432
                tunnel: w430 -> [w452]
                tunnel: [w451] -> w429
                frame #0 {
                  n160 = Concatenate Strings(w438, ".png" ("string")) -> (w437:string)
                  n161 = Build Path(base path=path "C:/Users/beck.to.beck/Documents/LabVIEW Data/BrBa/elements", name or relative path=w437) -> (appended path=w443:path)
                  n162 = call <vilib>:"Read PNG File.vi"("path to PNG file"=w443) -> ("image data"=w442:T6)  [unwired: 8 in, 2 out]
                  n163 = call "Empty Picture"() -> ("empty picture"=w444:picture)
                  n164 = call <vilib>:"Draw Flattened Pixmap.vi"("image data"=w442, "picture"=w444) -> ("new picture"=→"7":picture)  [unwired: 7 in]
                }
                frame #1 {
                  n165 = property on="7" class="Pict"("Visible"=TRUE) -> (error out=w450:errorcluster)  [unwired: 2 in, 1 out]
                  n166 = Bundle(w448, 240) -> (w446:cluster{i32, i32})  [unwired: 1 in]
                  n167 = property on="7" class="Pict"(error in=w450, "Position"=w446) -> (error out=w451:errorcluster)  [unwired: 1 in, 1 out]
                  n168 = Add(x=w448, y=w452) -> (x+y=w453:i32)
                }
              }
            }
            frame 8 {
              n169 = flat-sequence {
                tunnel: w459 -> [w463]
                tunnel: [w465] -> w460
                tunnel: w458 -> [w465]
                tunnel: w456 -> [w461]
                tunnel: [w461] -> w455
                tunnel: w460 -> [w478]
                tunnel: [w477] -> w457
                tunnel: w455 -> [w474]
                tunnel: [w476] -> w454
                frame #0 {
                  n170 = Concatenate Strings(w463, ".png" ("string")) -> (w462:string)
                  n171 = Build Path(base path=path "C:/Users/beck.to.beck/Documents/LabVIEW Data/BrBa/elements", name or relative path=w462) -> (appended path=w468:path)
                  n172 = call <vilib>:"Read PNG File.vi"("path to PNG file"=w468) -> ("image data"=w467:T6)  [unwired: 8 in, 2 out]
                  n173 = call "Empty Picture"() -> ("empty picture"=w469:picture)
                  n174 = call <vilib>:"Draw Flattened Pixmap.vi"("image data"=w467, "picture"=w469) -> ("new picture"=→"8":picture)  [unwired: 7 in]
                }
                frame #1 {
                  n175 = Bundle("y"=w474, 240) -> (w472:cluster{"y":i32, i32})  [unwired: 1 in]
                  n176 = property on="8" class="Pict"("Visible"=TRUE) -> (error out=w471:errorcluster)  [unwired: 2 in, 1 out]
                  n177 = property on="8" class="Pict"(error in=w471, "Position"=w472) -> (error out=w476:errorcluster)  [unwired: 1 in, 1 out]
                  n178 = Add(x=w474, y=w478) -> (x+y=w477:i32)
                }
              }
            }
            frame 9 {
              n179 = flat-sequence {
                tunnel: w485 -> [w489]
                tunnel: w484 -> [w486]
                tunnel: w482 -> [w487]
                tunnel: [w487] -> w481
                tunnel: [w486] -> w479
                tunnel: [w503] -> w483
                tunnel: w481 -> [w502]
                tunnel: [w501] -> w480
                tunnel: w479 -> [w499]
                frame #0 {
                  n180 = Concatenate Strings(w489, ".png" ("string")) -> (w488:string)
                  n181 = Build Path(base path=path "C:/Users/beck.to.beck/Documents/LabVIEW Data/BrBa/elements", name or relative path=w488) -> (appended path=w493:path)
                  n182 = call <vilib>:"Read PNG File.vi"("path to PNG file"=w493) -> ("image data"=w492:T6)  [unwired: 8 in, 2 out]
                  n183 = call "Empty Picture"() -> ("empty picture"=w494:picture)
                  n184 = call <vilib>:"Draw Flattened Pixmap.vi"("image data"=w492, "picture"=w494) -> ("new picture"=→"9":picture)  [unwired: 7 in]
                }
                frame #1 {
                  n185 = property on="9" class="Pict"("Visible"=TRUE) -> (error out=w496:errorcluster)  [unwired: 2 in, 1 out]
                  n186 = Bundle(w499, 240) -> (w497:cluster{i32, i32})  [unwired: 1 in]
                  n187 = property on="9" class="Pict"(error in=w496, "Position"=w497) -> (error out=w501:errorcluster)  [unwired: 1 in, 1 out]
                  n188 = Add(x=w499, y=w502) -> (x+y=w503:i32)
                }
              }
            }
          }
        }
        n189 = while {
          tunnel: w206 -> [_]
          tunnel: [w216] -> w205
          stop <- w217 stop-if-true
          n190 = event shown="[9] \"9\": Mouse Down" {
            selector: _ -> [_ _ _ _ _ _ _ _ _ _]
            dyn-events: _ -> [_ _ _ _ _ _ _ _ _ _]
            timeout: _ -> [_ _ _ _ _ _ _ _ _ _]
            tunnel: [TRUE TRUE TRUE TRUE TRUE TRUE TRUE TRUE TRUE TRUE] -> w217
            tunnel: [0 1 2 3 4 5 6 7 8 9] -> w216
            event "zero": Mouse Down {
              n191 = event-data() -> ()  [unwired: 1 in, 8 out]
            }
            event "1": Mouse Down {
              n192 = event-data() -> ()  [unwired: 1 in, 8 out]
            }
            event "2": Mouse Down {
              n193 = event-data() -> ()  [unwired: 1 in, 8 out]
            }
            event "3": Mouse Down {
              n194 = event-data() -> ()  [unwired: 1 in, 8 out]
            }
            event "4": Mouse Down {
              n195 = event-data() -> ()  [unwired: 1 in, 8 out]
            }
            event "5": Mouse Down {
              n196 = event-data() -> ()  [unwired: 1 in, 8 out]
            }
            event "6": Mouse Down {
              n197 = event-data() -> ()  [unwired: 1 in, 8 out]
            }
            event "7": Mouse Down {
              n198 = event-data() -> ()  [unwired: 1 in, 8 out]
            }
            event "8": Mouse Down {
              n199 = event-data() -> ()  [unwired: 1 in, 8 out]
            }
            event "9": Mouse Down {
              n200 = event-data() -> ()  [unwired: 1 in, 8 out]
            }
          }
        }
        n201 = Index Array(array=w204, index=w205) -> (element=w209:string)
        n202 = Bundle By Name(cluster=w211, "Chosen"=w209) -> (w210:T1)
      }
      frame "Selected" {
        w505 = T2[] [enum."PrepareToShowSelected"] items=["init", "idle", "Segregate", "Select", "Singles&Doubles", "SearchForElements", "Display", "PutInOrder", "OptionToSelect", "Selected", "ChooseByLuck", "PrepareToShowByLuck", "PrepareToShowSelected", "Show", "ShowOnce"] ("f")
        n203 = Unbundle By Name(w508) -> ("all 2"=w516:string[][][], "Cycles.Counter"=w517:i32, "WhichAndWhere"=w513:i32[])
        n204 = Decrement(x=w517) -> (x-1=w512:i32)
        n205 = Index Array(array=w513, index=w512) -> (element=w510:i32)
        n206 = Index Array(array=w516, index (dim 0)=w512) -> (element=w515:string[][])  [unwired: 2 in]
        n207 = Index Array(array=w515, index (row)=1) -> (element=w511:string[])  [unwired: 1 in]
        n208 = Index Array(array=w511, index=w510) -> (element=w509:string)
        n209 = To Lower Case(string=w509) -> (all lower case string=w504:string)
        n210 = Bundle By Name(cluster=w508, "Chosen"=w504) -> (w507:T1)
      }
      frame "ChooseByLuck" {
        w537 = T2[] [enum."PrepareToShowByLuck"] items=["init", "idle", "Segregate", "Select", "Singles&Doubles", "SearchForElements", "Display", "PutInOrder", "OptionToSelect", "Selected", "ChooseByLuck", "PrepareToShowByLuck", "PrepareToShowSelected", "Show", "ShowOnce"]
        n211 = Unbundle By Name(w536) -> ("SinglesInOrder"=w532:string[], "DoublesInOrder"=w524:string[], "all"=w531:string[][])
        n212 = Random Number (0-1)() -> (number: 0 to 1=w528:dbl)
        n213 = Array Size(array=w524) -> (size(s)=w523:i32)
        n214 = Multiply(x=w528, y=10.0) -> (x*y=w526:dbl)
        n215 = Not Equal?(x=w523, y=0) -> (x != y?=w521:bool)
        n216 = Greater?(x=w526, y=5.0) -> (0:w520:bool)
        n217 = Not And(1:w521, 2:w520) -> (0:w519:bool)
        n218 = case shown="True" w519 {
          tunnel: ["two" "one"] -> w518
          frame False {
          }
          frame True {
          }
        }
        n219 = Build Array(w532, w524) -> (w530:string[][])
        n220 = To Lower Case(string=w532) -> (all lower case string=w533:string[])
        n221 = Build Array (concatenate)(w531, w530) -> (w529:string[][])
        n222 = call "ByLuck.vi"("InOrder"=w533) -> ("ByLuck"=w539:string)  [unwired: 10 in]
        n223 = call "ByLuck.vi"("InOrder"=w524) -> ("ByLuck"=w538:string)  [unwired: 10 in]
        n224 = case shown="\"one\", Default" w518 {
          tunnel: w539 -> [_ w548]
          tunnel: w538 -> [w544 _]
          tunnel: [w545 w547] -> w534
          frame "two" {
            n225 = String Subset(string=w544, length (rest)=1 ("length (rest)")) -> (substring=w543:string)  [unwired: 1 in]
            n226 = To Lower Case(string=w543) -> (all lower case string=w545:string)
          }
          frame "one", Default {
            n227 = To Lower Case(string=w548) -> (all lower case string=w547:string)
          }
        }
        n228 = Bundle By Name(cluster=w536, "OptionForLuck"=w518, "ByLuck"=w534, "all"=w529) -> (w535:T1)
      }
      frame "PrepareToShowByLuck" {
        w566 = T2[] [enum."Select"] items=["init", "idle", "Segregate", "Select", "Singles&Doubles", "SearchForElements", "Display", "PutInOrder", "OptionToSelect", "Selected", "ChooseByLuck", "PrepareToShowByLuck", "PrepareToShowSelected", "Show", "ShowOnce"] ("f")
        w567 = T2[] [enum."Show"] items=["init", "idle", "Segregate", "Select", "Singles&Doubles", "SearchForElements", "Display", "PutInOrder", "OptionToSelect", "Selected", "ChooseByLuck", "PrepareToShowByLuck", "PrepareToShowSelected", "Show", "ShowOnce"]
        n229 = Unbundle By Name(w555) -> ("all 2"=w559:string[][][], "Array"=w561:T4, "AllLetters"=w556:string[], "ByLuck"=w565:string, "OptionForLuck"=w564:string)
        n230 = Bundle("AllLetters"=w556, "ByLuck"=w565, "OptionForLuck"=w564) -> (w562:T7)  [unwired: 1 in]
        n231 = Unbundle By Name(w555) -> ("SIndex"=w569:string[], "SinglesInOrder"=w575:string[], "DIndex"=w568:string[], "DoublesInOrder"=w574:string[])
        n232 = Build Array (concatenate)(w561, w562) -> (w563:T8)
        n233 = Bundle By Name(cluster=w555, "Array"=w563) -> (w558:T1)
        n234 = Build Array(w568, w574) -> (w572:string[][])
        n235 = Build Array(w569, w575) -> (w573:string[][])
        n236 = Transpose 2D Array(2D array=w573) -> (transposed array=w571:string[][])
        n237 = Transpose 2D Array(2D array=w572) -> (transposed array=w570:string[][])
        n238 = Build Array (concatenate)(w571, w570) -> (w560:string[][])
        n239 = Build Array (concatenate)(w559, w560) -> (w557:string[][][])
        n240 = Bundle By Name(cluster=w558, "all 2"=w557) -> (w552:T1)
        n241 = Unbundle By Name(w552) -> ("Cycles.Counter"=w551:i32, "Cycles.Laps"=w550:i32)
        n242 = Equal?(x=w551, y=w550) -> (x = y?=w549:bool)
        n243 = Select(t=w567, s=w549, f=w566) -> (s? t:f=w553:T2[])
      }
      frame "PrepareToShowSelected" {
        w590 = T2[] [enum."Select"] items=["init", "idle", "Segregate", "Select", "Singles&Doubles", "SearchForElements", "Display", "PutInOrder", "OptionToSelect", "Selected", "ChooseByLuck", "PrepareToShowByLuck", "PrepareToShowSelected", "Show", "ShowOnce"] ("f")
        w591 = T2[] [enum."Show"] items=["init", "idle", "Segregate", "Select", "Singles&Doubles", "SearchForElements", "Display", "PutInOrder", "OptionToSelect", "Selected", "ChooseByLuck", "PrepareToShowByLuck", "PrepareToShowSelected", "Show", "ShowOnce"]
        n244 = Unbundle By Name(w588) -> ("all 2"=w586:string[][][], "AllLetters"=w582:string[], "Chosen"=w581:string, "Array 2"=w580:T3, "Cycles.Counter"=w577:i32, "Cycles.Laps"=w576:i32)
        n245 = Equal?(x=w577, y=w576) -> (x = y?=w589:bool)
        n246 = Unbundle By Name(w588) -> ("SIndex"=w594:string[], "SinglesInOrder"=w600:string[], "DIndex"=w593:string[], "DoublesInOrder"=w599:string[])
        n247 = Bundle("AllLetters"=w582, "Chosen"=w581) -> (w578:cluster{"AllLetters":string[], "Chosen":string})  [unwired: 1 in]
        n248 = Build Array (concatenate)(w580, w578) -> (w579:T9)
        n249 = Bundle By Name(cluster=w588, "Array 2"=w579) -> (w585:T1)
        n250 = Build Array(w593, w599) -> (w597:string[][])
        n251 = Build Array(w594, w600) -> (w598:string[][])
        n252 = Transpose 2D Array(2D array=w598) -> (transposed array=w596:string[][])
        n253 = Transpose 2D Array(2D array=w597) -> (transposed array=w595:string[][])
        n254 = Build Array (concatenate)(w596, w595) -> (w587:string[][])
        n255 = Build Array (concatenate)(w586, w587) -> (w583:string[][][])
        n256 = Bundle By Name(cluster=w585, "all 2"=w583) -> (w584:T1)
        n257 = Select(t=w591, s=w589, f=w590) -> (s? t:f=w592:T2[])
      }
      frame "Show" {
        w613 = FALSE
        w617 = ""
        w620 = 0
        w626 = T2[] [enum."Display"] items=["init", "idle", "Segregate", "Select", "Singles&Doubles", "SearchForElements", "Display", "PutInOrder", "OptionToSelect", "Selected", "ChooseByLuck", "PrepareToShowByLuck", "PrepareToShowSelected", "Show", "ShowOnce"] ("f")
        n258 = Unbundle By Name(w622) -> ("Option"=w616:string, "Array"=w624:T4, "Array 2"=w623:T3, "ResultsAcumulado"=→"ResultsAcumulado":string[][][])
        n259 = control-ref of="Listbox"() -> (w625:refnum<vi>)
        n260 = Bundle By Name(cluster=w622, "Cycles.Laps"=w620, "Cycles.Counter"=w620, "Array"=T4 [], "Array 2"=T3 [], "ByLuck"=w617, "Chosen"=w617) -> (w621:T1)
        n261 = flat-sequence {
          tunnel: w625 -> [w631]
          tunnel: w624 -> [w630]
          tunnel: w623 -> [w629]
          tunnel: w616 -> [w628]
          tunnel: [w627] -> w615
          tunnel: w615 -> [w638]
          frame #0 {
            n262 = case shown="\"select\", Default" w628 {
              tunnel: w631 -> [w634 w637]
              tunnel: w630 -> [_ w636]
              tunnel: w629 -> [w633 _]
              tunnel: [w632 w635] -> w627
              frame "select", Default {
                n263 = call "new_show_outside.vi"("Multicolumn Listbox 2"=w634, "Array"=w633) -> ("max value"=w632:i32)  [unwired: 9 in]
              }
              frame "luck" {
                n264 = call "show3.vi"("Array"=w636, "Multicolumn Listbox 2"=w637) -> ("max value"=w635:i32)  [unwired: 7 in]
              }
            }
          }
          frame #1 {
            n265 = property on="Listbox" class="MCListbox (strict)"("NumCols"=w638) -> ()  [unwired: 2 in, 2 out]
          }
          frame #2 {
            n266 = invoke on="Listbox" class="MCListbox (strict)" method="Get Image"("image depth"=0 ("Image Depth"), "bg color"=u32 16448250) -> ("image data"=w641:T6)  [unwired: 4 in, 5 out]
            n267 = call <vilib>:"Write PNG File.vi"("image data"=w641, "path to PNG file"=path "C:/Users/beck.to.beck/Downloads/display.png" ("path to JPEG file")) -> ()  [unwired: 8 in, 2 out]
          }
        }
        n268 = property on="zero" class="Pict"(error in=w612, "Visible"=w613) -> (error out=w611:errorcluster)  [unwired: 1 in, 1 out]
        n269 = property on="1" class="Pict"(error in=w611, "Visible"=w613) -> (error out=w610:errorcluster)  [unwired: 1 in, 1 out]
        n270 = property on="2" class="Pict"(error in=w610, "Visible"=w613) -> (error out=w609:errorcluster)  [unwired: 1 in, 1 out]
        n271 = property on="3" class="Pict"(error in=w609, "Visible"=w613) -> (error out=w608:errorcluster)  [unwired: 1 in, 1 out]
        n272 = property on="4" class="Pict"(error in=w608, "Visible"=w613) -> (error out=w607:errorcluster)  [unwired: 1 in, 1 out]
        n273 = property on="5" class="Pict"(error in=w607, "Visible"=w613) -> (error out=w606:errorcluster)  [unwired: 1 in, 1 out]
        n274 = property on="6" class="Pict"(error in=w606, "Visible"=w613) -> (error out=w605:errorcluster)  [unwired: 1 in, 1 out]
        n275 = property on="7" class="Pict"(error in=w605, "Visible"=w613) -> (error out=w604:errorcluster)  [unwired: 1 in, 1 out]
        n276 = property on="8" class="Pict"(error in=w604, "Visible"=w613) -> (error out=w603:errorcluster)  [unwired: 1 in, 1 out]
        n277 = property on="9" class="Pict"(error in=w603, "Visible"=w613) -> (error out=w602:errorcluster)  [unwired: 1 in, 1 out]
      }
      frame "ShowOnce" {
        w647 = T2[] [enum."idle"] items=["init", "idle", "Segregate", "Select", "Singles&Doubles", "SearchForElements", "Display", "PutInOrder", "OptionToSelect", "Selected", "ChooseByLuck", "PrepareToShowByLuck", "PrepareToShowSelected", "Show", "ShowOnce"] ("f")
        n278 = Bundle By Name(cluster=w646, "ResultsAcumulado"=string[][][] []) -> (w645:T1)
      }
    }
  }
